vi "Get_VI_Icon.vi"(4 "BW Icon":T1, 6 "Color Icon":T1, 7 "Body Text":T2 {"Body Text Spec"."Alignment" items=["left", "center", "right"]}, 8 "error in (no error)":errorcluster, 9 "New VI template? (F)":bool) -> (0 "error out":errorcluster, 2 "VI Icon Data out":T5={"Text Visible?"=FALSE, "Text Opacity"=0, "Templ Visible?"=FALSE, "Templ Opacity"=0, "Relative Path from 1 to 2"=path "", "Image"=bytes[0], "All User Layers"=[], "Body Text"={"Line 1 text"="", "Line 2 text"="", "Line 3 text"="", "Line 4 text"="", "Line 1 color"=0, "Line 2 color"=0, "Line 3 color"=0, "Line 4 color"=0, "Body Text Spec"={"Font"="", "Alignment"=0, "Size"=3}, "Center text vertically"=FALSE, "Capitalize Text"=FALSE}} {"Body Text"."Body Text Spec"."Alignment" items=["left", "center", "right"]})   [LabVIEW 2020, in "lv_icon.lvlib"]
doc: "Get the LabVIEW Icon Data based on the inputs."
uses:
  <vilib>/LabVIEW Icon API/lv_icon/lv_icon.lvlib
  <vilib>/LabVIEW Icon API/lv_icon/Controls/LabVIEW Icon Stored Information.ctl
  <vilib>/LabVIEW Icon API/lv_icon/Classes/Layer/Layer.lvclass
  <vilib>/LabVIEW Icon API/lv_icon/Controls/BodyText.ctl
  <vilib>/LabVIEW Icon API/lv_icon/Controls/Font.ctl
  <vilib>/LabVIEW Icon API/lv_icon/Controls/Alignment.ctl
  <vilib>/picture/picture.llb/imagedata.ctl
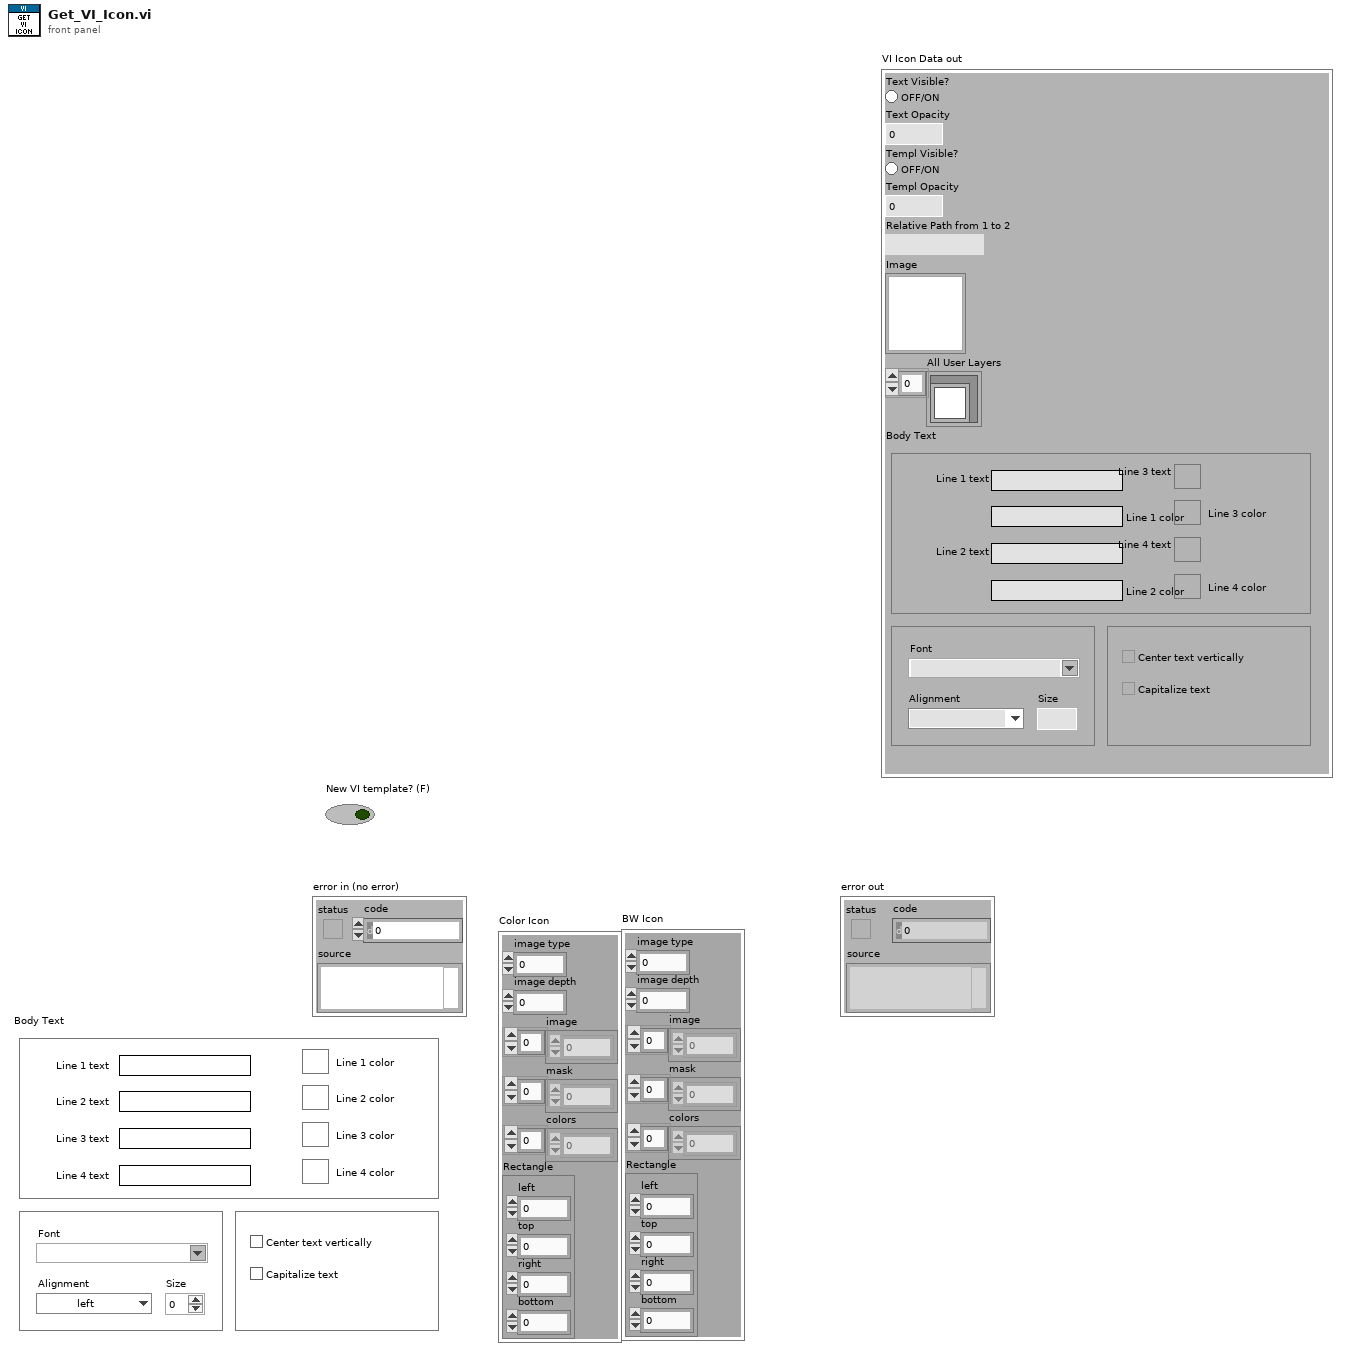
[diagram p1: front panel]
types:
  T1 = typedef "imagedata.ctl" = cluster{"image type":i32, "image depth":i32, "image":u8[], "mask":u8[], "colors":u32[], "Rectangle":cluster{"left":i16, "top":i16, "right":i16, "bottom":i16}}
  T2 = typedef "BodyText.ctl" = cluster{"Line 1 text":string, "Line 2 text":string, "Line 3 text":string, "Line 4 text":string, "Line 1 color":u32, "Line 2 color":u32, "Line 3 color":u32, "Line 4 color":u32, "Body Text Spec":cluster{"Font":T3, "Alignment":T4, "Size":u8}, "Center text vertically":bool, "Capitalize Text":bool}
  T3 = typedef "Font.ctl" = string
  T4 = typedef "Alignment.ctl" = u16
  T5 = typedef "LabVIEW Icon Stored Information.ctl" = cluster{"Text Visible?":bool, "Text Opacity":u8, "Templ Visible?":bool, "Templ Opacity":u8, "Relative Path from 1 to 2":path, "Image":picture, "All User Layers":refnum<class "Layer.lvclass">[], "Body Text":T2}
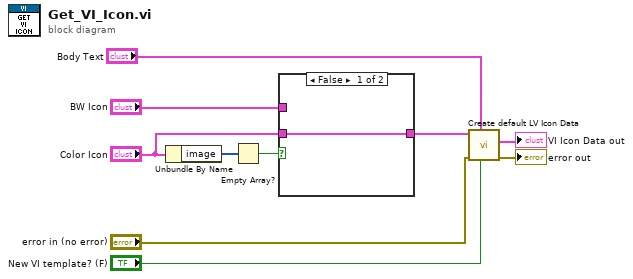
[diagram p0: block diagram]
diagram:
  n1 = Unbundle By Name("Color Icon") -> ("image"=w7:u8[])
  n2 = Empty Array?(array=w7) -> (empty?=w6:bool)
  n3 = case shown="False" w6 {
    tunnel: "Color Icon" -> [w11 _]
    tunnel: [w11 w12] -> w5
    tunnel: "BW Icon" -> [_ w12]
    frame False {
    }
    frame True {
    }
  }
  n4 = call <vilib>:"Create default LV Icon Data.vi"("New VI template? (F)"="New VI template? (F)", "Body Text"="Body Text", "error in"="error in (no error)", "Pic Data in"=w5) -> ("error out"=→"error out":errorcluster, "VI Icon Data out"=→"VI Icon Data out":T5)  [unwired: 2 in, 4 out]
